vi "Route Sync Pulse.vi"(8 "error in (no error)":errorcluster, 10 "sync pulse rtsi line":string, 11 "fpga interfaces in":refnum<k20>[](array[refnum])) -> (0 "error out":errorcluster, 3 "fpga interfaces out":refnum<k20>[](array[refnum]))   [LabVIEW 2021]
uses:
  <resource>/objmgr/sessionReference.rc
  <instrlib>/FlexRIO/API/Host/v1/NI FlexRIO API v1.lvlib
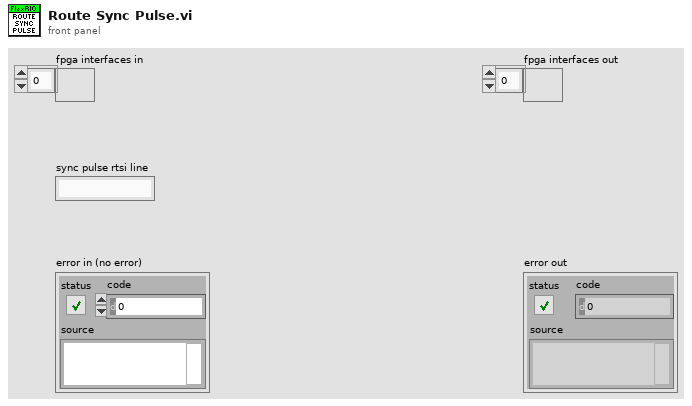
[diagram p1: front panel]
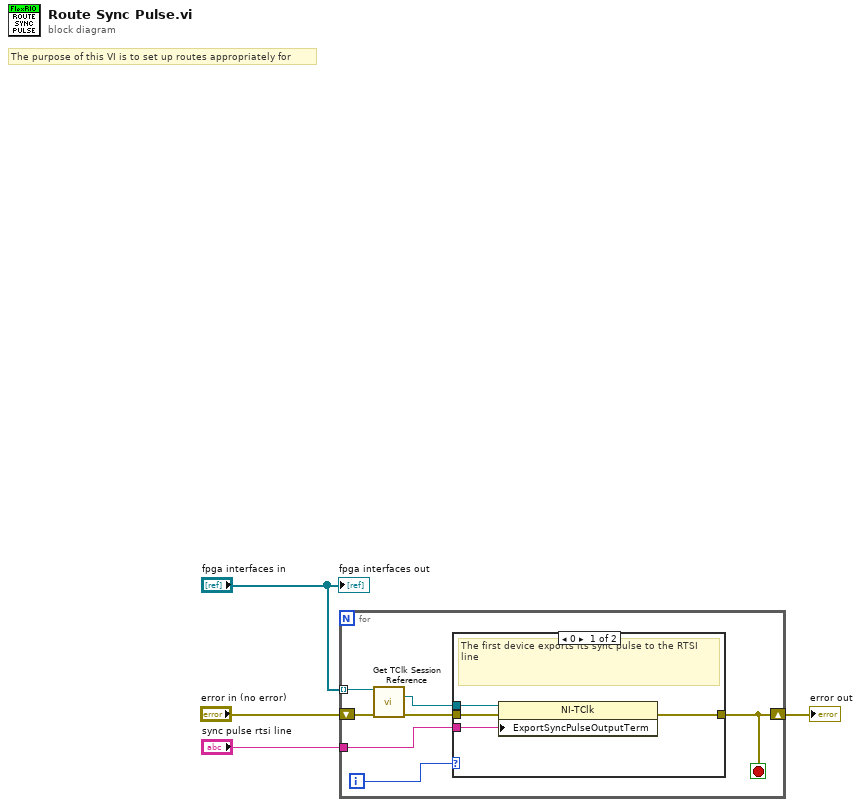
[diagram p0: block diagram]
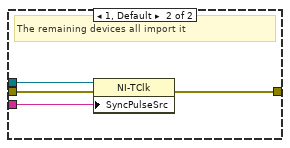
[diagram p2: hidden frame]
diagram:
  # "The purpose of this VI is to set up routes appropriately for"
  n1 = for {
    tunnel: "fpga interfaces in" -> [w6] mode=indexing
    tunnel: "sync pulse rtsi line" -> [w10]
    shift-right: [w9] -> w1
    shift-left: "error in (no error)" -> [w8]
    i -> [w11]
    stop <- w9 stop-if-true
    n2 = call <instrlib>:"Get TClk Session Reference.vi"("fpga interface in"=w6, "error in"=w8) -> ("tclk session reference"=w5:refnum<k20>, "error out"=w7:errorcluster)  [unwired: 11 in, 1 out]
    n3 = case shown="0" w11 {
      tunnel: w5 -> [w15 w19]
      tunnel: w10 -> [w14 w18]
      tunnel: w7 -> [w13 w17]
      tunnel: [w12 w16] -> w9
      frame 0 {
        # "The first device exports its sync pulse to the RTSI line"
        n4 = property class="NI-TClk"(reference=w15, error in=w13, "ExportSyncPulseOutputTerm"=w14) -> (error out=w12:errorcluster)  [unwired: 1 out]
      }
      frame 1, Default {
        # "The remaining devices all import it"
        n5 = property class="NI-TClk"(reference=w19, error in=w17, "SyncPulseSrc"=w18) -> (error out=w16:errorcluster)  [unwired: 1 out]
      }
    }
  }
  "error out" <- w1
  "fpga interfaces out" <- "fpga interfaces in"
